vi "m10.wf.samplingInfo.vi"(10 "Duration (s)":dbl, 11 "Fs (Hz)":dbl min=0.0) -> (3 "sampling info":cluster{"Fs":dbl, "#s":dbl} {"Fs" format="%.2p"})   [LabVIEW 2009]
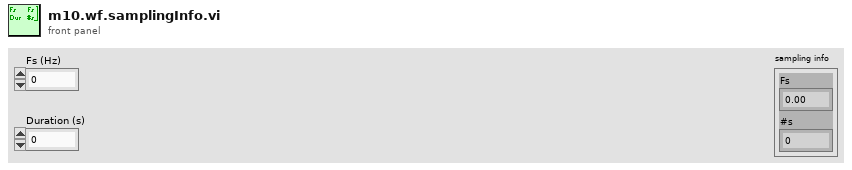
[diagram p1: front panel]
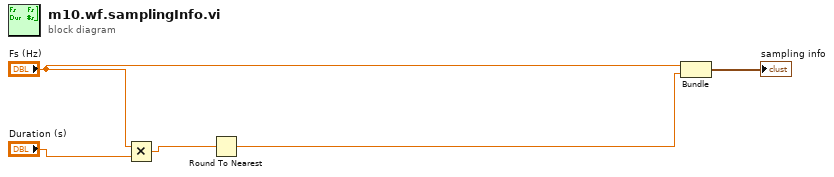
[diagram p0: block diagram]
diagram:
  n1 = Multiply(x="Fs (Hz)", y="Duration (s)") -> (x*y=w2:dbl)
  n2 = Round To Nearest(number=w2) -> (nearest integer value=w1:dbl)
  n3 = Bundle("Fs (Hz)"="Fs (Hz)", w1) -> (→"sampling info":cluster{"Fs (Hz)":dbl, dbl})  [unwired: 1 in]
